vi "TiePie.Lst.LstOpenDevice.vi"(8 "error in (no error)":errorcluster, 9 "dwDeviceType":u32, 10 "dwId":u32, 11 "dwIdKind":u32) -> (0 "error out":errorcluster, 3 "GenHandle":T1)   [LabVIEW 2014, in "LVTiePie.lvlib"]
uses:
  LVTiePie.lvlib
  TiePie.Gen.handle.ctl
  bin/libtiepie.dll
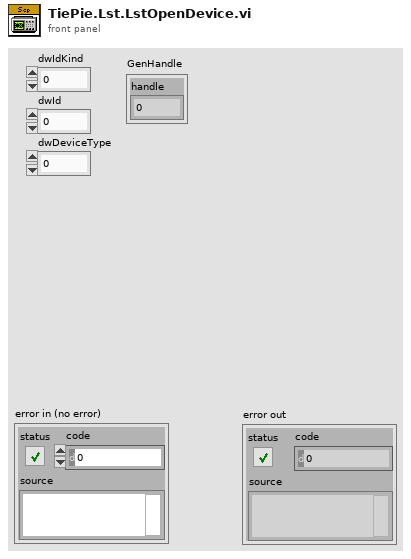
[diagram p1: front panel]
types:
  T1 = typedef "TiePie.Gen.handle.ctl" = cluster{"handle":u32}
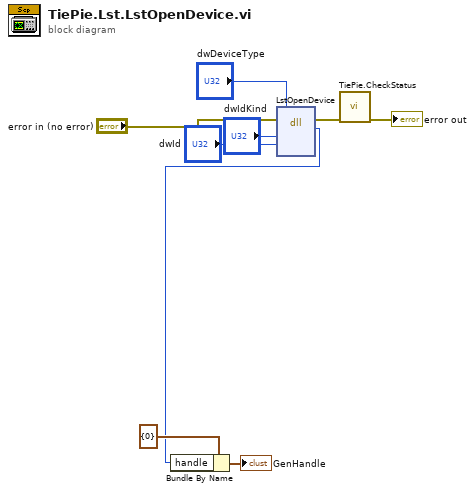
[diagram p0: block diagram]
diagram:
  n1 = dll-call lib="C:/Users/mbirski/Desktop/PAN/LabVEW/Tie Pie/bin/libtiepie.dll" fn="LstOpenDevice"(error in="error in (no error)", "dwIdKind"="dwIdKind", "dwId"="dwId", "dwDeviceType"="dwDeviceType") -> (error out=w8:errorcluster, "handle"=w4:u32)  [unwired: 5 in, 1 out]
  n2 = Bundle By Name(cluster=T1 {"handle"=0} ("GenHandle"), "handle"=w4) -> (→"GenHandle":T1)
  n3 = call "TiePie.CheckStatus.vi"("error in (no error)"=w8) -> ("error out"=→"error out":errorcluster)  [unwired: 10 in]
